vi "read_FE_memory_n.vi"(2 "execute":bool, 11 "error in (no error)":errorcluster) -> (4 "function return":string, 6 "CRC OK":bool=TRUE, 8 "length 4":i32, 10 "I2C FE mem":string="Single shunt, R(Z1), 1kohm, S/N: 4\u0000                                                                                                                                                                                                                                                                                                                                                                                                                                                                                                                                                                                     ...", 15 "error out":errorcluster)   [LabVIEW 2017, in "ZBOX_IS.lvlib"]
uses:
  ZBOX_IS.lvlib
panel:
  out "function return 2":string
  in  "read cycles":i32=88
  out "length 3":i32=90
  out "uLPtr 4":u32[](array[numeric])
  out "ulValue 2":u32
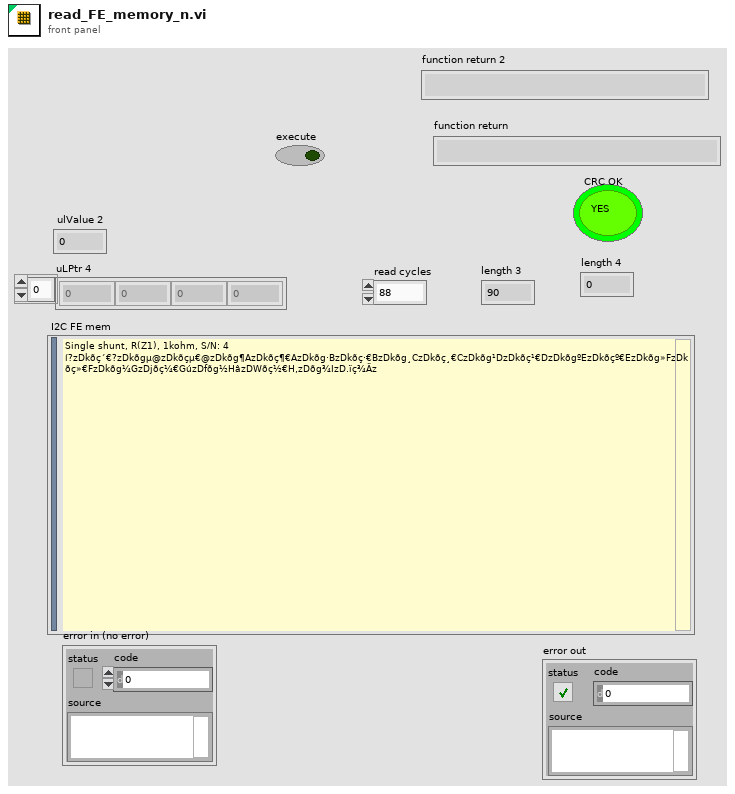
[diagram p1: front panel]
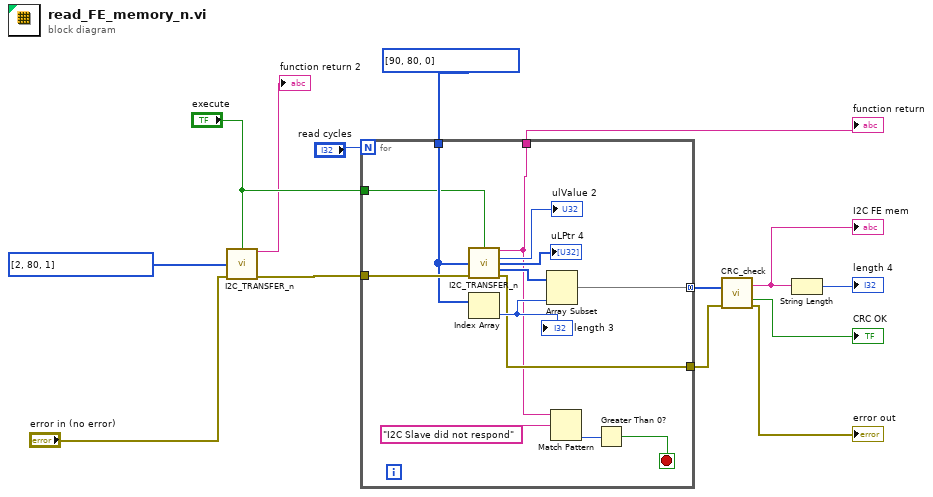
[diagram p0: block diagram]
diagram:
  n1 = call "I2C_TRANSFER_n.vi"("execute"="execute", "uLPtr"=u32[] [2, 80, 1] ("i2c read"), "error in (no error)"="error in (no error)") -> ("function return"=→"function return 2":string, "error out"=w8:errorcluster)  [unwired: 8 in, 3 out]
  n2 = for {
    N: "read cycles" -> [_]
    tunnel: [w27] -> w11 mode=concatenating
    tunnel: w8 -> [w22]
    tunnel: u32[] [90, 80, 0] ("i2c read") -> [w21]
    tunnel: [w18] -> w6
    tunnel: [w20] -> w4
    tunnel: "execute" -> [w19]
    stop <- w15 stop-if-true
    n3 = call "I2C_TRANSFER_n.vi"("execute"=w19, "uLPtr"=w21, "error in (no error)"=w22) -> ("function return"=w18:string, "ulValue"=→"ulValue 2":u32, "uLPtr"=→"uLPtr 4":u32[], "BytePtr"=w23:u8[], "error out"=w20:errorcluster)  [unwired: 8 in]
    n4 = Index Array(array=w21) -> (element=w26:u32)  [unwired: 1 in]
    "length 3" <- w26
    n5 = Array Subset(array=w23, length=w26) -> (w27:u8[])  [unwired: 1 in]
    n6 = Match Pattern(string=w18, regular expression="I2C Slave did not respond" ("function return")) -> (offset past match=w16:i32)  [unwired: 1 in, 3 out]
    n7 = Greater Than 0?(x=w16) -> (x > 0?=w15:bool)
  }
  "function return" <- w6
  n8 = call "CRC_check.vi"("IN"=w11, "error in (no error)"=w4) -> ("bin from I2C"=w13:string, "CRC"=→"CRC OK":bool, "error out"=→"error out":errorcluster)  [unwired: 9 in, 2 out]
  "I2C FE mem" <- w13
  n9 = String Length(string=w13) -> (length=→"length 4":i32)
